vi "Motor_V_Control.vi"() -> ()   [LabVIEW 2014]
uses:
  <vilib>/Simulation/Scripting/Companion Diagram/SimConfigNode/SimParams.ctl
  <vilib>/Simulation/Scripting/Companion Diagram/SimConfigNode/_simSolvers.ctl
  <vilib>/Simulation/Implementation/Shared/SIMSCR Execution Mode.ctl
  <vilib>/Simulation/Param Hierarchy/Typedefs/SIMPH Param Control Actions.ctl
  <vilib>/Simulation/Implementation/Shared/NILVSim_ParamChanged.vi
  <vilib>/Simulation/Implementation/Shared/NILVSIM_BeginStep.vi
  <vilib>/Simulation/DataSources/Implementation/NILVSim Step.llb/SIM Step (scalar).vi
  <vilib>/Simulation/SignalDisplay/Implementation/NILVSim Time Waveform.llb/SIM Time Waveform (scalar).vi
  <vilib>/Simulation/SignalArithmetic/Implementation/NILVSim Gain.llb/SIM Gain (scalar).vi
  <vilib>/Simulation/Implementation/Shared/NILVSim_Manager.vi
  <vilib>/Utility/error.llb/Clear Errors.vi
  <vilib>/Simulation/Implementation/Shared/NILVSim_FinalizeModel.vi
  <vilib>/Simulation/Implementation/Shared/SIM Unbundle Sim Info.vi
  <vilib>/Simulation/Implementation/Shared/NILVSim_Initialize.vi
  <vilib>/Simulation/Utility/Implementation/NILVSim Get Time and IsAcceptedStep.vi
  <vilib>/addons/control/pid/pid.llb/PID.vi
  <vilib>/addons/control/pid/pid.llb/PID (DBL).vi
  <vilib>/Simulation/Implementation/Shared/SIMSH Read Queue.vi
  <vilib>/Simulation/Implementation/Shared/NILVSim_GetModelError.vi
  <vilib>/Simulation/Implementation/Shared/SIM Bundle Sim Info.vi
  <vilib>/Simulation/Scripting/Companion Diagram/SimConfigNode/SimDog.xnode
  Motor_subsys.vi
  <vilib>/Simulation/Implementation/XNodeFramework/SimXNode/SimX.xnode
  <vilib>/addons/control/pid/NI_PID_pid.lvlib
  <vilib>/Simulation/Implementation/Shared/NI_SIM_Implementation.lvlib
panel:
  out "Duty Cycle":waveform(dbl)(graph)={"t0"=timestamp(1 s since 1904-01-01), "dt"=1.0, "Y"=[0.3095791268704745]}
  in  "Desired Velocity":dbl=300.0
  in  "PID gains":T1={"proportional gain (Kc)"=0.0006, "integral time (Ti, min)"=0.0005, "derivative time (Td, min)"=0.0} {"derivative time (Td, min)" format="%.3f"; "integral time (Ti, min)" format="%.3e"; "proportional gain (Kc)" format="%.3e"}
  out "d_theta":dbl=299.9997462601454
  out "Angular Velocity":waveform(dbl)(graph)={"t0"=timestamp(1 s since 1904-01-01), "dt"=1.0, "Y"=[299.9997462601454]}
  in  "R [ohm]":dbl=5.0
  in  "B [Nms]":dbl=1.65e-05
  in  "K [Nm/Amp]":dbl=0.0208
  in  "J [kg*m^2]":dbl=3.129e-06
  in  "L [H]":dbl=0.00018
  # "Tune the value of Inductance"
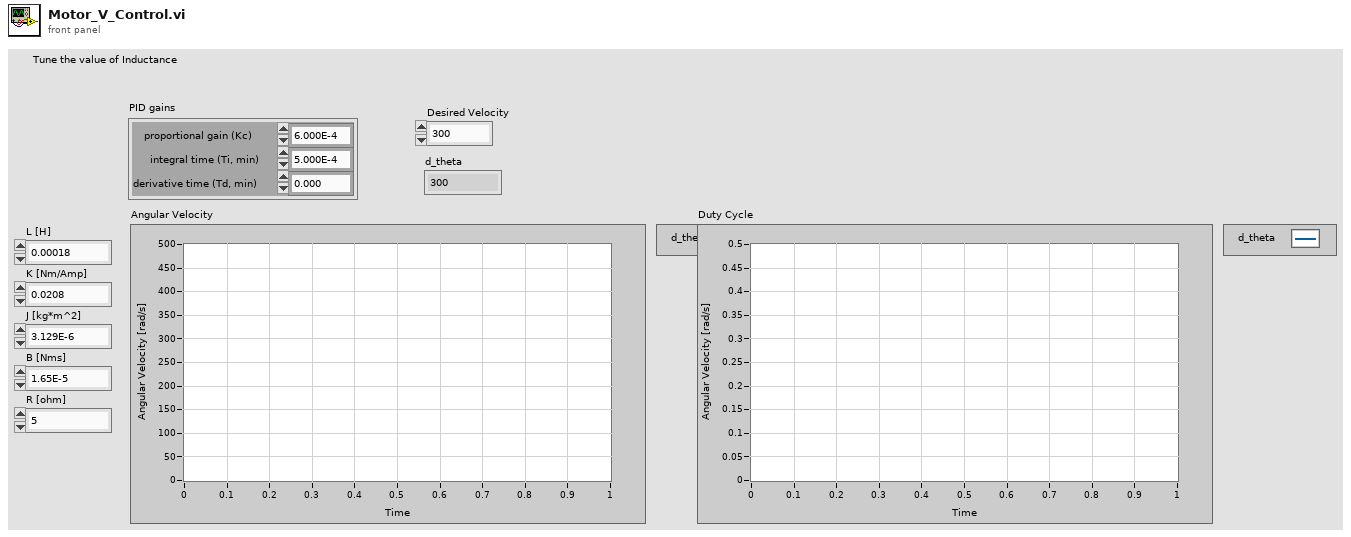
[diagram p1: front panel]
types:
  T1 = cluster{"proportional gain (Kc)":dbl, "integral time (Ti, min)":dbl, "derivative time (Td, min)":dbl}
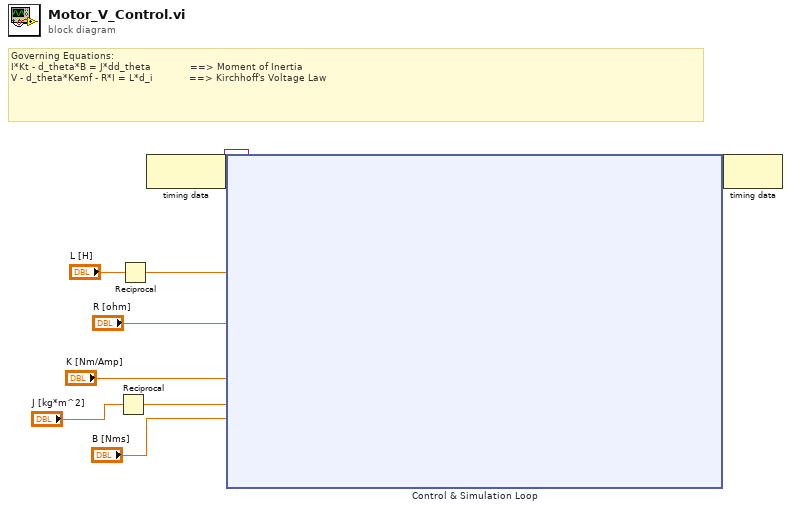
[diagram p0: block diagram]
diagram:
  # "Governing Equations: \nI*Kt - d_theta*B = J*dd_theta             ==> Moment of Inertia\nV - d_theta*Kemf - R*I = L*d_i            ==> Kirchhoff's Voltage Law"
  n1 = Reciprocal(x="J [kg*m^2]") -> (1/x=w4:dbl)
  n2 = Reciprocal(x="L [H]") -> (1/x=w6:dbl)
  n3 = node-c288() -> (w9:variant)  [unwired: 1 in]
  n4 = node-c254 "Control & Simulation Loop"(w9, w6, w4, "K [Nm/Amp]", "B [Nms]", "R [ohm]") -> (w8:variant)
  n5 = node-c288(w8) -> ()  [unwired: 1 out]
